vi "Config Drive Pipeline Command.vi"(8 "Command Info In":T2, 10 "Drive Conditions":T1) -> (0 "Command Info Out":T2)   [LabVIEW 2025]
uses:
  <vilib>/Rock Robotics/WPI/Framework/Command Status Info.ctl
  <vilib>/Rock Robotics/WPI/Framework/Completion Status.ctl
  <vilib>/Rock Robotics/WPI/Framework/Completion Notifier.ctl
  Framework/Drive Conditions.ctl
  Framework/Robot Global Data.vi
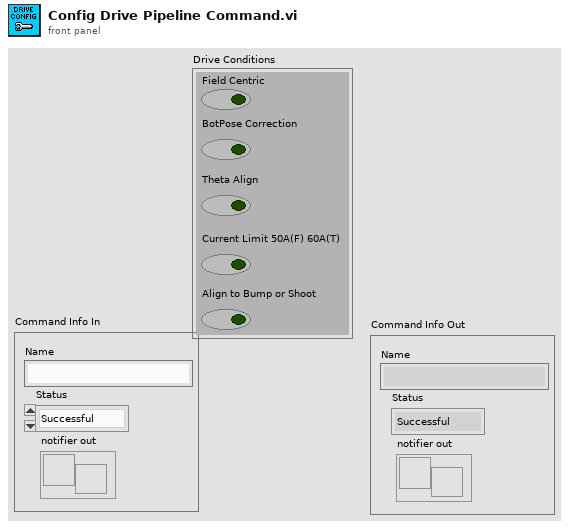
[diagram p1: front panel]
types:
  T1 = typedef "Drive Conditions.ctl" = cluster{"Field Centric":bool, "BotPose Correction":bool, "Theta Align":bool, "Current Limit 50A(F) 60A(T)":bool, "Align to Bump or Shoot":bool}
  T2 = typedef "Command Status Info.ctl" = cluster{"Name":string, "Status":T3, "notifier out":T4}
  T3 = typedef "Completion Status.ctl" = enum16{"Successful", "Aborted", "Incomplete"}
  T4 = typedef "Completion Notifier.ctl" = refnum<notifier>
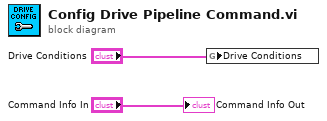
[diagram p0: block diagram]
diagram:
  n1 = global write "Robot Global Data.vi" "Drive Conditions"("Drive Conditions") -> ()
  "Command Info Out" <- "Command Info In"
